vi "DJ Interface.vi"(10 "Owning VI":refnum<vi>, 11 "Shutdown Event":refnum<user-event>) -> ()   [LabVIEW 2018, in "User Interface.lvlib"]
doc: "Main control interface to Dataflow DJ. Also handles all keyboard shortcuts.\n\n<b>Execution System:</b> User Interface"
uses:
  User Interface.lvlib
  Custom Graphics/Slide.Vert.ctl
  Custom Graphics/LED.Red.16px.ctl
  Custom Graphics/Slide.Horiz.ctl
  Custom Graphics/Slide.PlaybackPosition.ctl
  Custom Graphics/WaveformGraph.WaveformDisplay.ctl
  Custom Graphics/Knob.276px_Hole.ctl
  Custom Graphics/Button.Large.ctl
  Custom Graphics/PictRing.DeckLabel.ctl
  Custom Graphics/Button.Small.ctl
  <vilib>/Utility/miscctls.llb/LVCursorListTypeDef.ctl
  Audio Processing/Value Properties.ctl
  Messaging/Message Cluster.ctl
  Controls/Keyboard Shortcut.ctl
  1bc07e46-b0f0-44a4-aabd-5c34d242854a.vi
  Messaging/Messaging.lvlib
  user32.dll
  Audio Processing/Audio Processing.lvlib
panel:
  in  "Mixer.Channel2.EQFilter":dbl(knob) scale=-1.025..1.025
  in  "Mixer.Channel1.EQFilter":dbl(knob) scale=-1.025..1.025
  in  "Deck2.DragDropPath":path
  in  "Deck1.DragDropPath":path
  in  "Deck1.Pitch":T1 scale=30.0..-30.0
  in  "Deck2.PitchBendUp":T2
  in  "Deck2.PitchBendDown":T2
  in  "Mixer.Channel2.HeadphoneOutput":T2
  in  "Mixer.Channel1.HeadphoneOutput":T2
  in  "Deck1.PitchBendUp":T2
  in  "Deck1.PitchBendDown":T2
  in  "Deck2.Reverse":T3
  in  "Deck2.Backspin":T3
  in  "Deck2.Brake":T3
  in  "Deck2.Cue3":T3
  in  "Deck2.Cue2":T3
  in  "Deck2.Cue1":T3
  in  "Deck2.Play":T3
  in  "Deck1.Cue3":T3
  in  "Deck1.Cue2":T3
  in  "Deck1.Reverse":T3
  in  "Deck1.Backspin":T3
  in  "Deck1.Cue1":T3
  out "Deck2.Time":string
  in  "Deck2.PlaybackPosition":T4 scale=0.0..7050240.0
  out "Deck2.Waveform":T5
  out "Deck2.BPM":string
  out "Deck1.BPM":string
  in  "Mixer.Headphones":dbl(knob)=1.0 scale=0.0..1.0
  in  "Deck1.Brake":T3
  in  "Mixer.Channel2.Effect3.Value2":dbl(knob) scale=0.0..1.0
  in  "Mixer.Channel2.Effect3.Enable":T6
  in  "Mixer.Channel2.Effect3.Value1":dbl(knob) scale=0.0..1.0
  in  "Mixer.Channel2.Effect2.Enable":T6
  in  "Mixer.Channel2.Effect2.Value1":dbl(knob)=1.0 step=1.0 scale=1.0..20.0
  in  "Mixer.Channel2.Effect2.Value2":dbl(knob)=16.0 step=1.0 scale=0.0..16.0
  in  "Mixer.Channel2.Effect1.Enable":T6
  in  "Mixer.Channel2.Effect1.Value1":dbl(knob) scale=0.0..1.0
  in  "Mixer.Channel2.Effect1.Value2":dbl(knob) scale=0.001..0.1
  in  "Mixer.Channel1.Effect3.Value2":dbl(knob) scale=0.0..1.0
  in  "Mixer.Channel1.Effect3.Enable":T6
  in  "Mixer.Channel1.Effect3.Value1":dbl(knob) scale=0.0..1.0
  out "Mixer.Channel2.LevelIndicator":u8(slide) scale=0.0..20.0
  out "Mixer.Channel1.LevelIndicator":u8(slide) scale=0.0..20.0
  in  "Mixer.Channel1.Effect2.Enable":T6
  in  "Mixer.Channel1.Effect2.Value1":dbl(knob)=1.0 step=1.0 scale=1.0..20.0
  in  "Mixer.Channel1.Effect2.Value2":dbl(knob)=16.0 step=1.0 scale=0.0..16.0
  in  "Mixer.Channel1.Effect1.Enable":T6
  in  "Deck1.Play":T3
  in  "Mixer.Master":dbl(knob)=1.0 scale=0.0..1.0
  in  "Deck1.Jogwheel":T7 scale=0.0..79380.0
  in  "Mixer.Channel1.Effect1.Value1":dbl(knob) scale=0.0..1.0
  in  "Mixer.Channel1.Effect1.Value2":dbl(knob) scale=0.001..0.1
  in  "Deck2.Pitch":T1 scale=30.0..-30.0
  out "Deck2.Title":string
  out "Deck1.Time":string
  out "Deck1.Title":string
  in  "Deck2.Jogwheel":T7 scale=0.0..79380.0
  in  "Mixer.Channel2.Level":T1=1.0 scale=0.0..1.0
  in  "Mixer.Channel2.EQHighKill":T6
  in  "Mixer.Channel2.EQMidKill":T6
  in  "Mixer.Channel2.EQLow":dbl(knob)=1.0 scale=0.0..2.0
  in  "Mixer.Channel2.EQMid":dbl(knob)=1.0 scale=0.0..2.0
  in  "Mixer.Channel2.EQHigh":dbl(knob)=1.0 scale=0.0..2.0
  in  "Mixer.Channel2.EQLowKill":T6
  in  "Mixer.Channel2.Gain":dbl(knob)=1.0 scale=0.0..2.0
  in  "Mixer.Crossfader":T8 scale=-1.0..1.0
  in  "Mixer.Channel1.Level":T1=1.0 scale=0.0..1.0
  in  "Mixer.Channel1.EQHighKill":T6
  in  "Mixer.Channel1.EQMidKill":T6
  in  "Mixer.Channel1.EQLow":dbl(knob)=1.0 scale=0.0..2.0
  in  "Mixer.Channel1.EQMid":dbl(knob)=1.0 scale=0.0..2.0
  in  "Mixer.Channel1.EQHigh":dbl(knob)=1.0 scale=0.0..2.0
  in  "Mixer.Channel1.EQLowKill":T6
  in  "Mixer.Channel1.Gain":dbl(knob)=1.0 scale=0.0..2.0
  in  "Deck1.PlaybackPosition":T4 scale=0.0..7050240.0
  out "Deck1.Waveform":T5
  out "Deck1.JogwheelLabel":T9
  out "Deck2.JogwheelLabel":T9
  # "GAIN"
  # "MASTER"
  # "PHONES"
  # "GAIN"
  # "FLANGER"
  # "FLANGER"
  # "AMOUNT"
  # "SPEED"
  # "AMOUNT"
  # "SPEED"
  # "CRUSHER"
  # "CRUSHER"
  # "DECIMATION"
  # "BIT DEPTH"
  # "DECIMATION"
  # "BIT DEPTH"
  # "ECHO"
  # "ECHO"
  # "AMOUNT"
  # "DELAY"
  # "AMOUNT"
  # "DELAY"
  # "DECK 1\nCUE"
  # "DECK 2\nCUE"
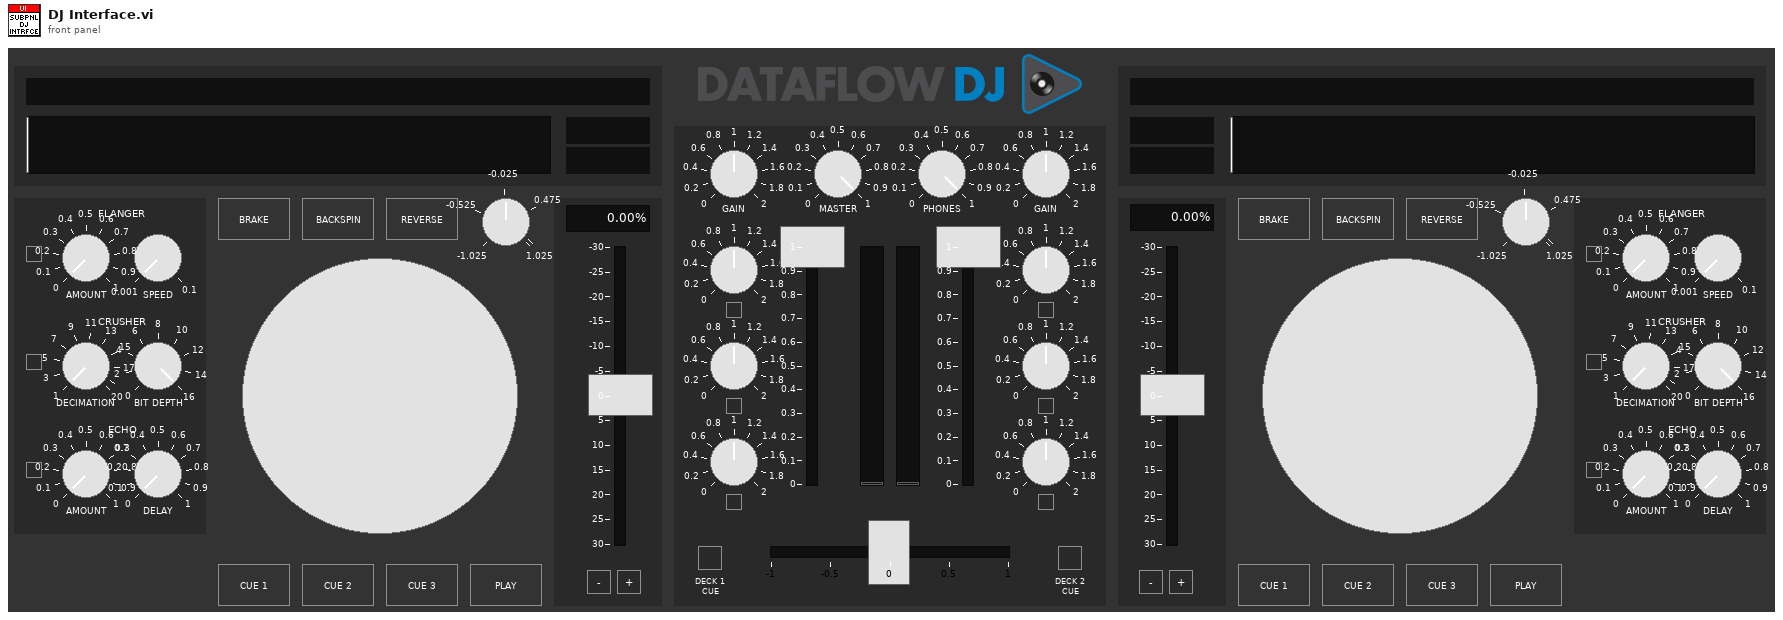
[diagram p1: front panel]
types:
  T1 = typedef "User Interface.lvlib/Slide.Vert.ctl" = dbl
  T2 = typedef "User Interface.lvlib/Button.Small.ctl" = bool
  T3 = typedef "User Interface.lvlib/Button.Large.ctl" = bool
  T4 = typedef "User Interface.lvlib/Slide.PlaybackPosition.ctl" = i32
  T5 = typedef "User Interface.lvlib/WaveformGraph.WaveformDisplay.ctl" = dbl[][]
  T6 = typedef "User Interface.lvlib/LED.Red.16px.ctl" = bool
  T7 = typedef "User Interface.lvlib/Knob.276px_Hole.ctl" = i32
  T8 = typedef "User Interface.lvlib/Slide.Horiz.ctl" = dbl
  T9 = typedef "User Interface.lvlib/PictRing.DeckLabel.ctl" = u16
  T10 = typedef "LVCursorListTypeDef.ctl" = cluster{"Name":string, "Color":u32, "Style":u8, "Point Style":u8, "Name Visible":bool, "Allow Drag":bool, "Cursor Mode":u32, "Plot":i32, "Index":i32, "Position":cluster{"X":dbl, "Y":dbl}, "X Scale":u32, "Y Scale":u32, "Watch Plots":i32[], "Watch All Plots":bool, "Plot Area":i32, "Label Offset":cluster{"X":dbl, "Y":dbl}}[]
  T11 = typedef "Keyboard Shortcut.ctl" = cluster{"Keystroke":string, "Message Queue":string, "Event":string, "Target":string, "Data":variant}
  T12 = typedef "Audio Processing.lvlib/Value Properties.ctl" = cluster{"Lower":dbl, "Upper":dbl}
  T13 = typedef "Messaging.lvlib/Message Cluster.ctl" = cluster{"Event":string, "Source":string, "Target":string, "Data":variant}
  T14 = cluster{"type":i32, "KEYBDINPUT":cluster{"dx":i32, "dy":i32, "mouseData":i32, "dwFlags":i32, "time":i32, "dwExtraInfo":u32}}
  T15 = typedef "eventvkey.ctl" = enum16{"ASCII", "Enter", "Return", "Shift", "Ctrl", "Alt", "Cmd", "Opt", "Caps", "NumLock", "Clear", "Break", "Up", "Down", "Left", "Right", "Insert", "Delete", "Home", "End", "PageUp", "PageDown", "Escape", "Help", "Pause", "ScrollLock", "F1", "F2", "F3", "F4", "F5", "F6", "F7", "F8", "F9", "F10", "F11", "F12", "F13", "F14", "F15", "F16", "F17", "F18", "F19", "F20", "F21", "F22", "F23", "F24", "Play", "VolumeUp", "VolumeDown", "Mute", "Two Byte Char"}
  T16 = cluster{"Shift":bool, "Ctrl":bool, "Alt":bool, "Cmd":bool, "Opt":bool}
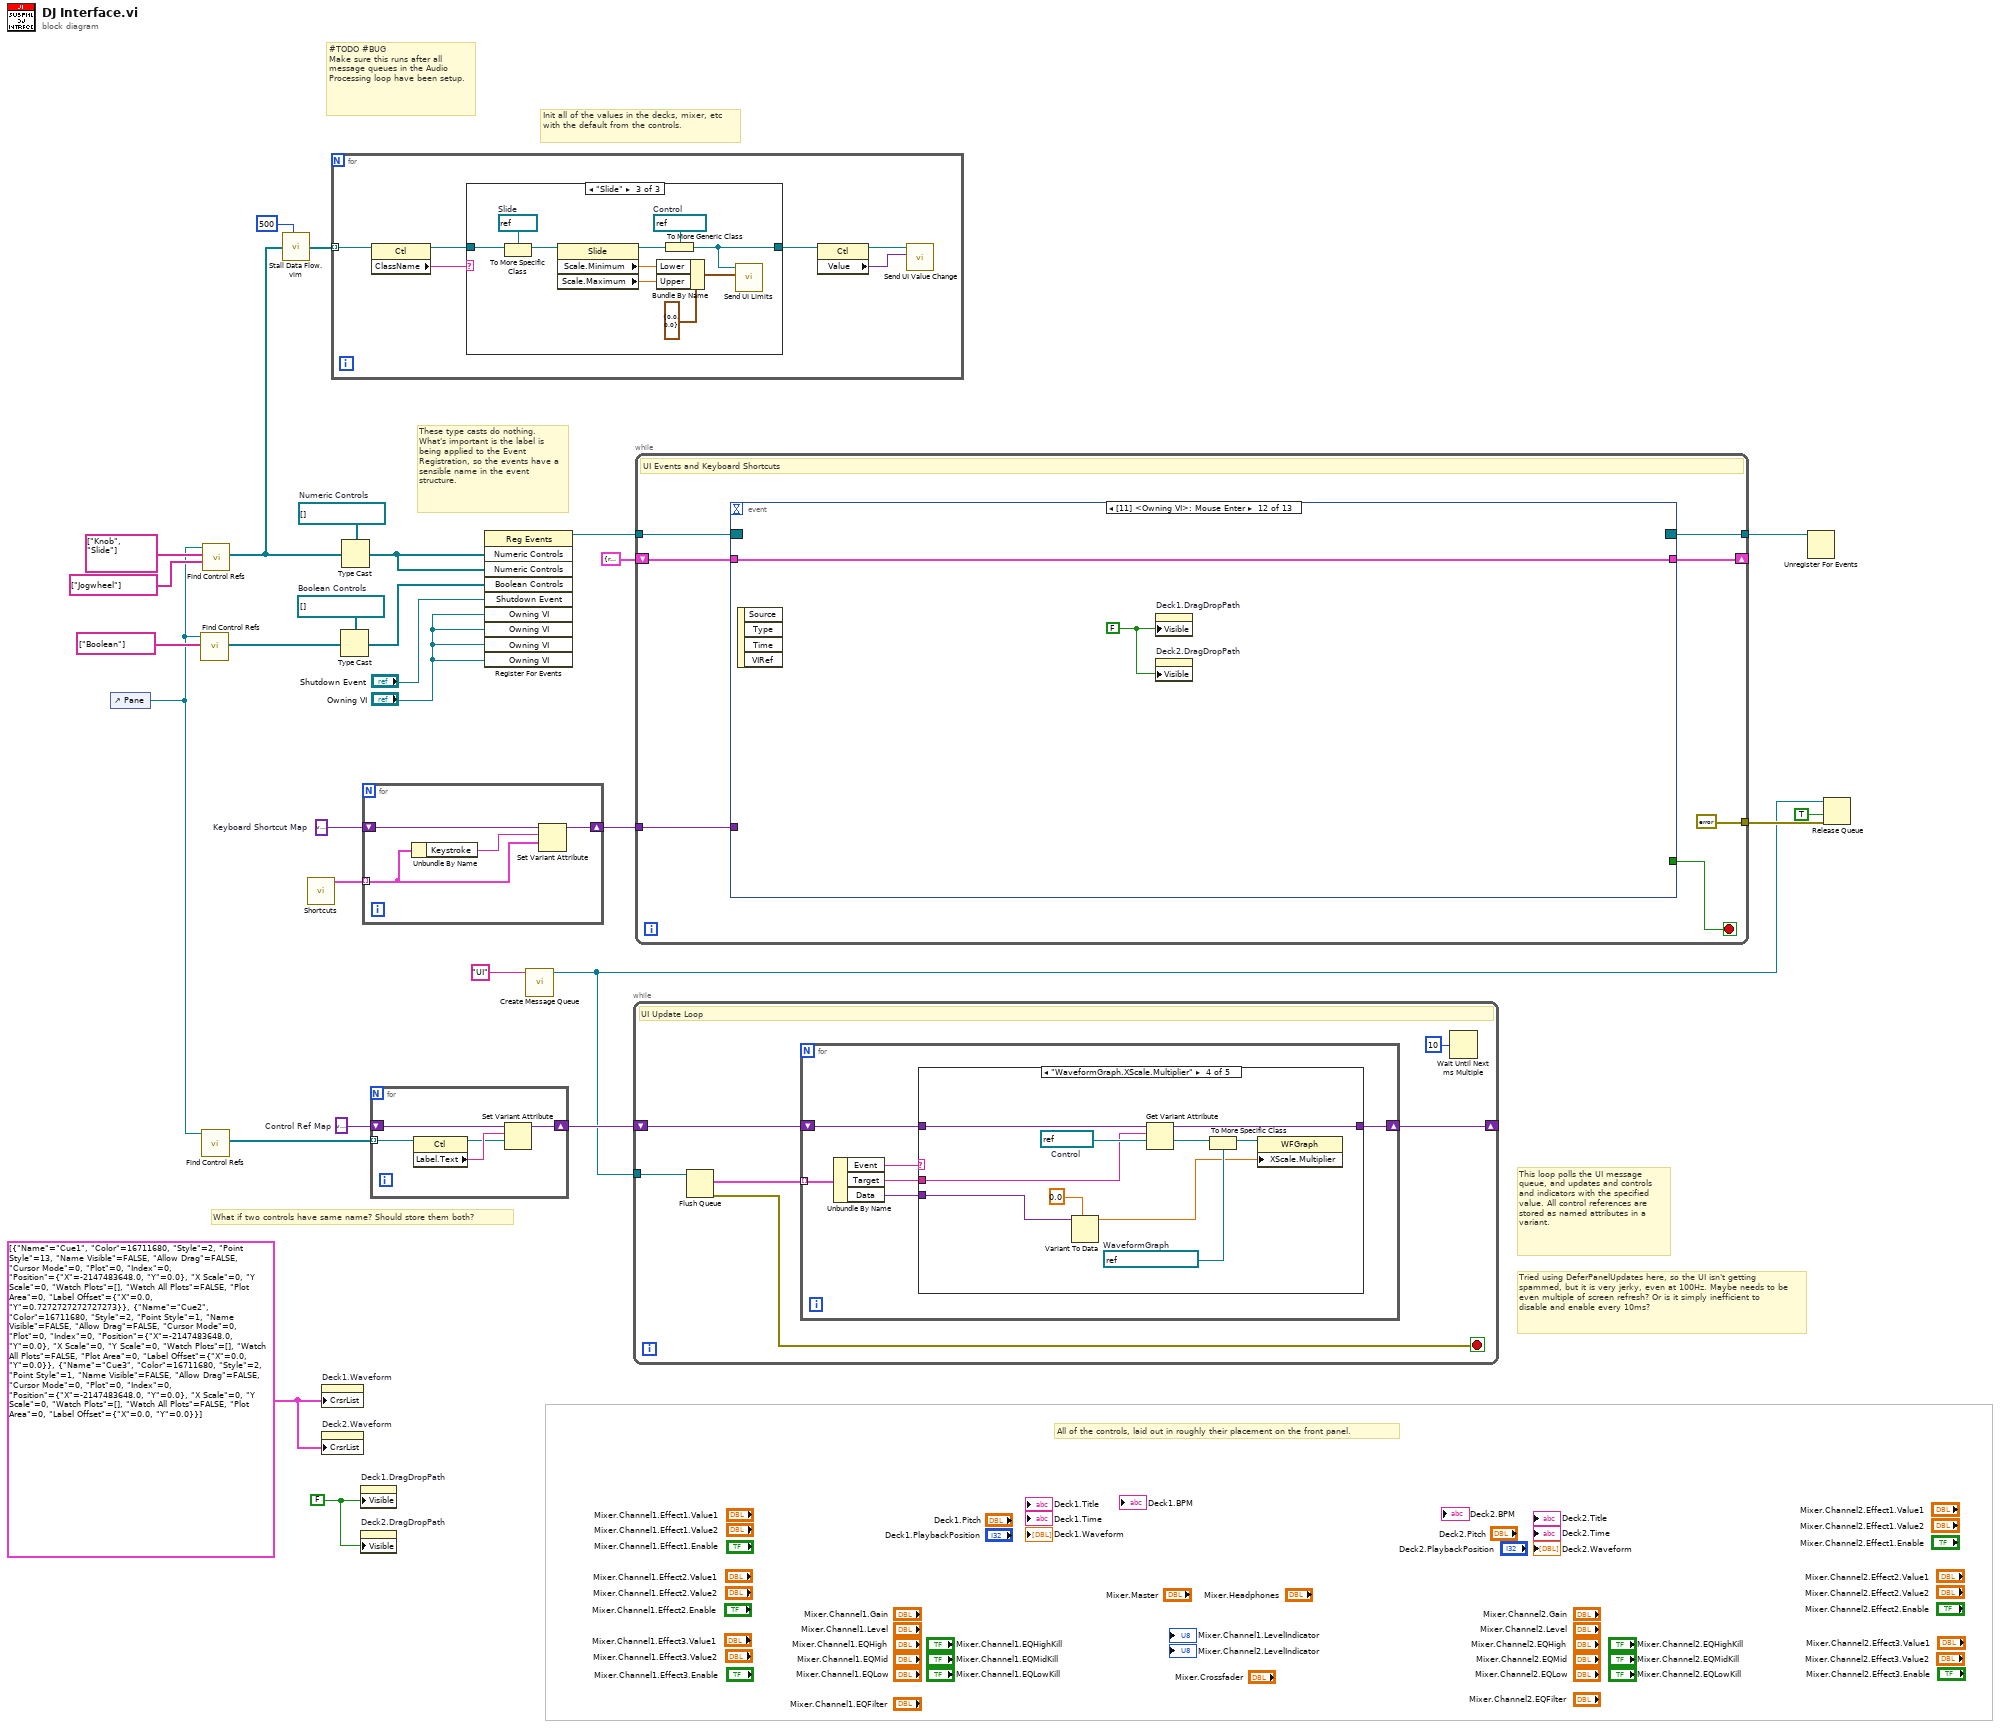
[diagram p0: block diagram]
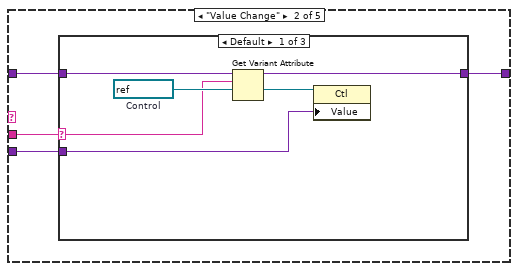
[diagram p3: hidden frame]
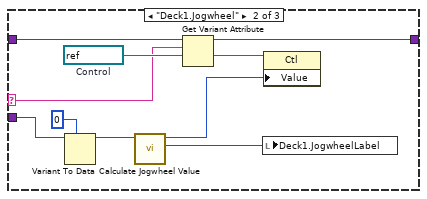
[diagram p4: hidden frame]
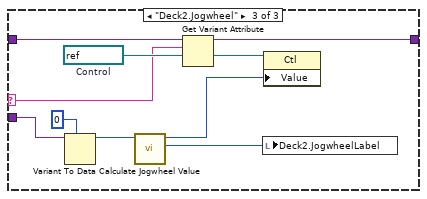
[diagram p5: hidden frame]
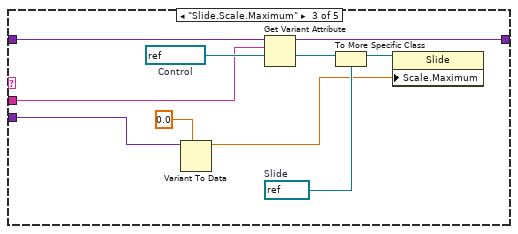
[diagram p6: hidden frame]
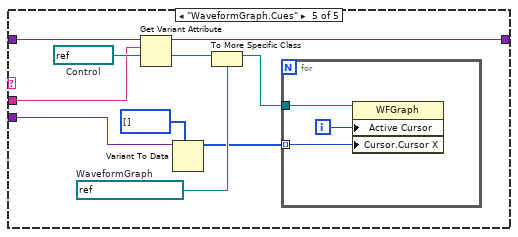
[diagram p7: hidden frame]
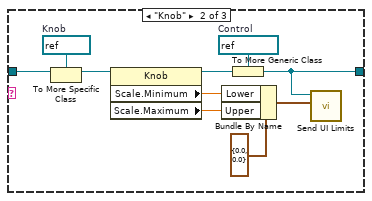
[diagram p9: hidden frame]
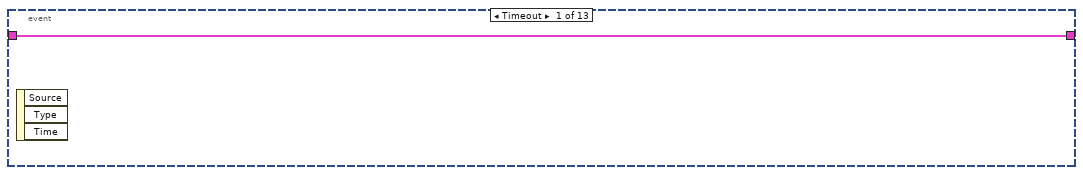
[diagram p10: hidden frame]
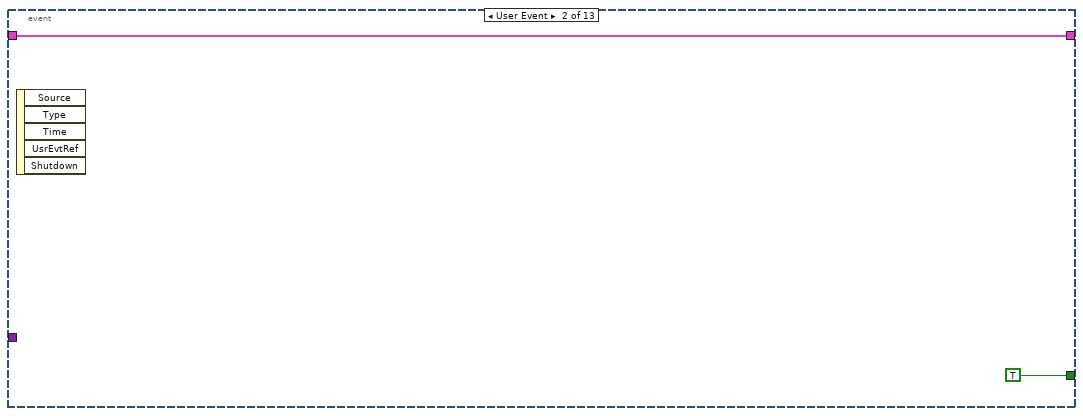
[diagram p11: hidden frame]
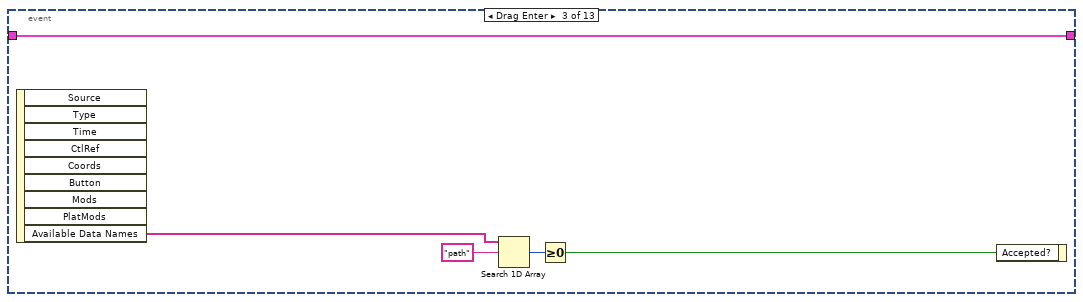
[diagram p12: hidden frame]
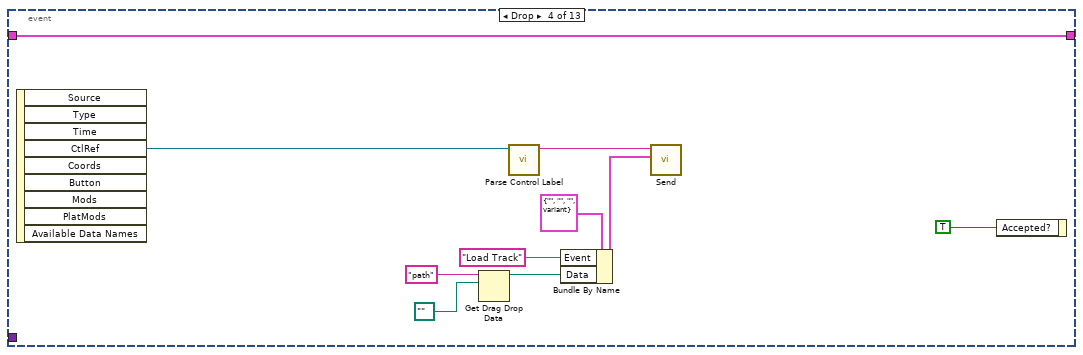
[diagram p13: hidden frame]
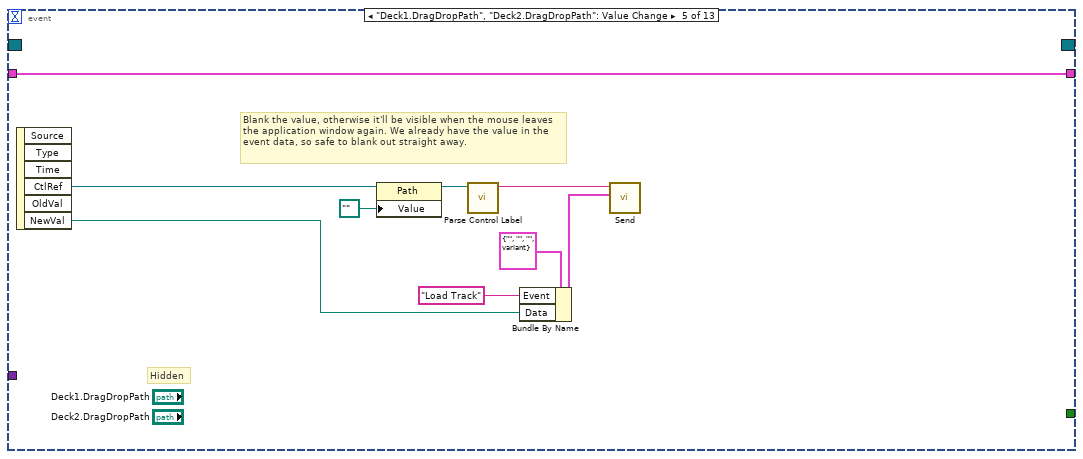
[diagram p14: hidden frame]
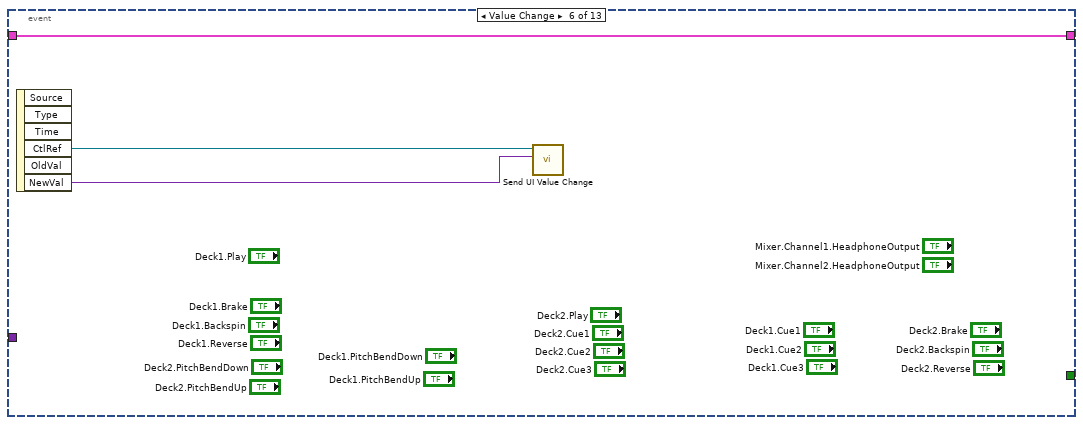
[diagram p15: hidden frame]
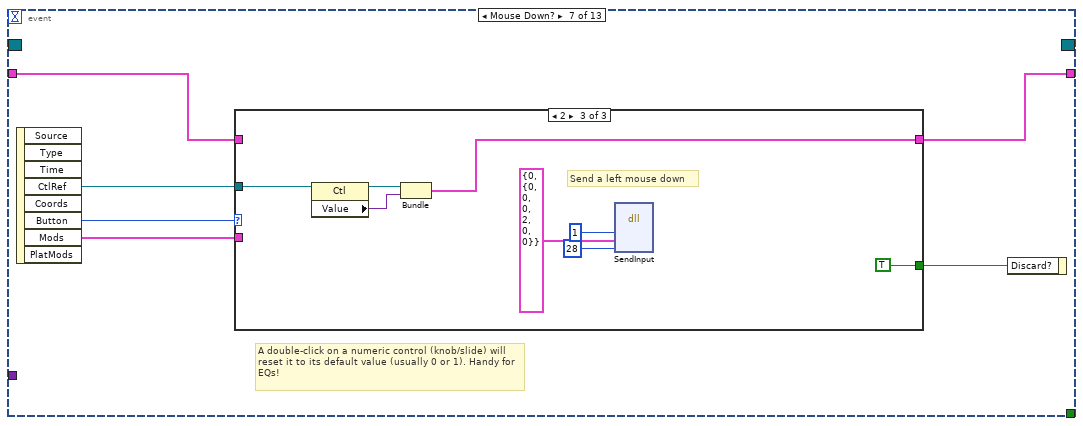
[diagram p16: hidden frame]
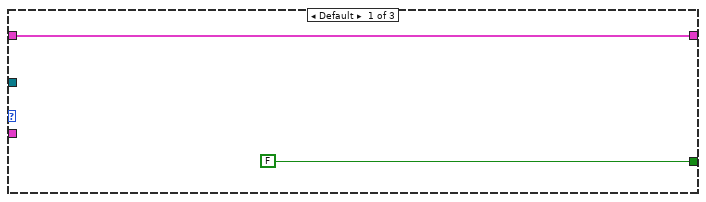
[diagram p17: hidden frame]
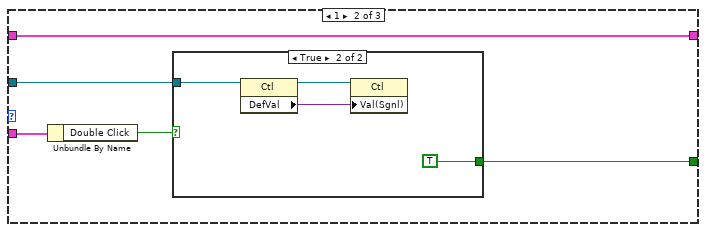
[diagram p18: hidden frame]
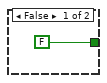
[diagram p19: hidden frame]
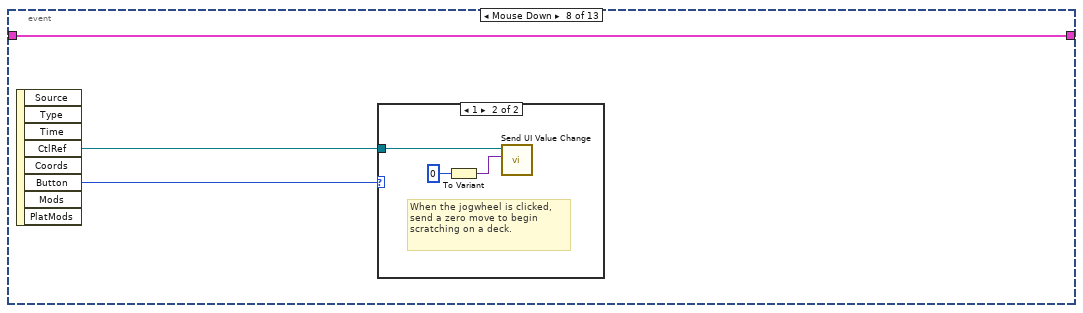
[diagram p20: hidden frame]
diagram:
  w4 = FALSE ("Visible")
  w6 = T10 [{"Name"="Cue1", "Color"=16711680, "Style"=2, "Point Style"=13, "Name Visible"=FALSE, "Allow Drag"=FALSE, "Cursor Mode"=0, "Plot"=0, "Index"=0, "Position"={"X"=-2147483648.0, "Y"=0.0}, "X Scale"=0, "Y Scale"=0, "Watch Plots"=[], "Watch All Plots"=FALSE, "Plot Area"=0, "Label Offset"={"X"=0.0, "Y"=0.7272727272727273}}, {"Name"="Cue2", "Color"=16711680, "Style"=2, "Point Style"=1, "Name Visible"=FALSE, "Allow Drag"=FALSE, "Cursor Mode"=0, "Plot"=0, "Index"=0, "Position"={"X"=-2147483648.0, "Y"=0.0}, "X Scale"=0, "Y Scale"=0, "Watch Plots"=[], "Watch All Plots"=FALSE, "Plot Area"=0, "Label Offset"={"X"=0.0, "Y"=0.0}}, {"Name"="Cue3", "Color"=16711680, "Style"=2, "Point Style"=1, "Name Visible"=FALSE, "Allow Drag"=FALSE, "Cursor Mode"=0, "Plot"=0, "Index"=0, "Position"={"X"=-2147483648.0, "Y"=0.0}, "X Scale"=0, "Y Scale"=0, "Watch Plots"=[], "Watch All Plots"=FALSE, "Plot Area"=0, "Label Offset"={"X"=0.0, "Y"=0.0}}] ("Cursor List")
  w21 = variant  # Keyboard Shortcut Map
  w24 = variant  # Control Ref Map
  w28 = refnum<vi>[] []  # Boolean Controls
  w27 = refnum<vi>[] []  # Numeric Controls
  # "Init all of the values in the decks, mixer, etc with the default from the controls."
  # "#TODO #BUG\nMake sure this runs after all message queues in the Audio Processing loop have been setup."
  # "What if two controls have same name? Should store them both?"
  # "All of the controls, laid out in roughly their placement on the front panel."
  # "This loop polls the UI message queue, and updates and controls and indicators with the specified value. All control references are stored as named attributes in a variant."
  # "Tried using DeferPanelUpdates here, so the UI isn't getting spammed, but it is very jerky, even at 100Hz. Maybe needs to be even multiple of screen refresh? Or is it simply inefficient to disable and enable every 10ms?"
  # "These type casts do nothing. What's important is the label is being applied to the Event Registration, so the events have a sensible name in the event structure."
  n1 = control-ref of="Pane"() -> (w10:refnum<vi>)
  n2 = call "Find Control Refs.vi"("Control Types"=string[] ["Boolean"], "Pane Reference In"=w10) -> ("Control Refs"=w11:refnum<vi>[])  [unwired: 8 in, 1 out]
  n3 = call "Find Control Refs.vi"("Pane Reference In"=w10) -> ("Control Refs"=w9:refnum<vi>[])  [unwired: 9 in, 1 out]
  n4 = call "Find Control Refs.vi"("Label.Text Filter"=string[] ["Jogwheel"], "Control Types"=string[] ["Knob", "Slide"], "Pane Reference In"=w10) -> ("Control Refs"=w3:refnum<vi>[])  [unwired: 7 in, 1 out]
  n5 = call "Stall Data Flow.vim"("value in"=w3, "milliseconds to wait"=u32 500) -> ("value out"=w2:refnum<vi>[])  [unwired: 1 out]
  n6 = call "Shortcuts.vi"() -> ("Keyboard Shortcuts"=w19:T11[])  [unwired: 11 in]
  n7 = property on="Deck1.Waveform" class="WFGraph (strict)"("CrsrList"=w6) -> ()  [unwired: 2 in, 2 out]
  n8 = property on="Deck2.Waveform" class="WFGraph (strict)"("CrsrList"=w6) -> ()  [unwired: 2 in, 2 out]
  n9 = for {
    tunnel: w2 -> [w31] mode=indexing
    n10 = property class="Ctl"(reference=w31) -> (reference out=w32:refnum<vi>, "ClassName"=w30:string)  [unwired: 1 in, 1 out]
    n11 = case shown="\"Slide\"" w30 {
      tunnel: [w36 w41 w48] -> w33
      tunnel: w32 -> [w36 w46 w56]
      frame Default {
      }
      frame "Knob" {
        w42 = refnum<vi> refnum  # Control
        w45 = refnum<vi> refnum  # Knob
        n12 = To More Specific Class(target class=w45, reference=w46) -> (specific class reference=w44:refnum<vi>)  [unwired: 1 in, 1 out]
        n13 = property class="Knob"(reference=w44) -> (reference out=w43:refnum<vi>, "Scale.Minimum"=w39:dbl, "Scale.Maximum"=w38:dbl)  [unwired: 1 in, 1 out]
        n14 = Bundle By Name(cluster=T12 {"Lower"=0.0, "Upper"=0.0} ("Value Properties"), "Lower"=w39, "Upper"=w38) -> (w37:T12)
        n15 = To More Generic Class(target class=w42, reference=w43) -> (generic class reference=w41:refnum<vi>)
        n16 = call "Send UI Limits.vi"("Data"=w37, "CtlRef"=w41) -> ()  [unwired: 10 in]
      }
      frame "Slide" {
        w49 = refnum<vi> refnum  # Control
        w55 = refnum<vi> refnum  # Slide
        n17 = To More Specific Class(target class=w55, reference=w56) -> (specific class reference=w54:refnum<vi>)  [unwired: 1 in, 1 out]
        n18 = property class="Slide"(reference=w54) -> (reference out=w50:refnum<vi>, "Scale.Minimum"=w53:dbl, "Scale.Maximum"=w52:dbl)  [unwired: 1 in, 1 out]
        n19 = Bundle By Name(cluster=T12 {"Lower"=0.0, "Upper"=0.0} ("Value Properties"), "Lower"=w53, "Upper"=w52) -> (w51:T12)
        n20 = To More Generic Class(target class=w49, reference=w50) -> (generic class reference=w48:refnum<vi>)
        n21 = call "Send UI Limits.vi"("Data"=w51, "CtlRef"=w48) -> ()  [unwired: 10 in]
      }
    }
    n22 = property class="Ctl"(reference=w33) -> (reference out=w34:refnum<vi>, "Value"=w35:variant)  [unwired: 1 in, 1 out]
    n23 = call "Send UI Value Change.vi"("Data"=w35, "CtlRef"=w34) -> ()  [unwired: 10 in]
  }
  n24 = Type Cast(type=w28, x=w11) -> (*(type *) &x=w25:refnum<vi>[])
  n25 = Type Cast(type=w27, x=w3) -> (*(type *) &x=w8:refnum<vi>[])
  n26 = property on="Deck1.DragDropPath" class="Path"("Visible"=w4) -> ()  [unwired: 2 in, 2 out]
  n27 = property on="Deck2.DragDropPath" class="Path"("Visible"=w4) -> ()  [unwired: 2 in, 2 out]
  n28 = for {
    shift-right: [w59] -> w20
    shift-left: w21 -> [w60]
    tunnel: w19 -> [w57] mode=indexing
    n29 = Unbundle By Name(w57) -> ("Keystroke"=w58:string)
    n30 = Set Variant Attribute(Variant=w60, name=w58, value=w57) -> (Variant out=w59:variant)  [unwired: 1 in, 2 out]
  }
  n31 = for {
    shift-right: [w64] -> w23
    shift-left: w24 -> [w65]
    tunnel: w9 -> [w63] mode=indexing
    n32 = property class="Ctl"(reference=w63) -> (reference out=w61:refnum<vi>, "Label.Text"=w62:string)  [unwired: 1 in, 1 out]
    n33 = Set Variant Attribute(Variant=w65, name=w62, value=w61) -> (Variant out=w64:variant)  [unwired: 1 in, 2 out]
  }
  n34 = register-events(w8, w8, w25, "Shutdown Event", "Owning VI", "Owning VI", "Owning VI", "Owning VI") -> (reference out=w29:refnum<event-registration>)  [unwired: 2 in, 1 out]
  n35 = call "Create Message Queue.vi"("Queue Name"="UI") -> ("queue out"=w15:refnum<queue>)  [unwired: 9 in, 1 out]
  n36 = while {
    tunnel: w15 -> [w69]
    shift-right: [w70] -> _
    shift-left: w23 -> [w71]
    stop <- w67 stop-if-true
    # "UI Update Loop"
    n37 = Flush Queue(queue=w69) -> (remaining elements=w66:T13[], error out=w67:errorcluster)  [unwired: 1 in, 1 out]
    n38 = for {
      shift-right: [w76] -> w70
      shift-left: w71 -> [w77]
      tunnel: w66 -> [w72] mode=indexing
      n39 = Unbundle By Name(w72) -> ("Event"=w75:string, "Target"=w73:string, "Data"=w74:variant)
      n40 = case shown="\"WaveformGraph.XScale.Multiplier\"" w75 {
        tunnel: w77 -> [w78 w82 w118 w128 w138]
        tunnel: w73 -> [_ w79 w115 w125 w135]
        tunnel: [w78 w81 w116 w126 w136] -> w76
        tunnel: w74 -> [_ w80 w110 w120 w130]
        frame Default {
        }
        frame "Value Change" {
          n41 = case shown="Default" w79 {
            selector: w79 -> [w83 w94 w104]
            tunnel: w82 -> [w88 w98 w108]
            tunnel: [w85 w95 w105] -> w81
            tunnel: w80 -> [w84 w93 w103]
            frame Default {
              w87 = refnum<vi> refnum  # Control
              n42 = Get Variant Attribute(Variant=w88, name=w83, default value (empty Variant)=w87) -> (duplicate Variant=w85:variant, value=w86:refnum<vi>)  [unwired: 1 in, 2 out]
              n43 = property class="Ctl"(reference=w86, "Value"=w84) -> ()  [unwired: 1 in, 2 out]
            }
            frame "Deck1.Jogwheel" {
              w97 = refnum<vi> refnum  # Control
              n44 = Variant To Data(type=0 ("y"), Variant=w93) -> (data=w91:i32)  [unwired: 1 in, 1 out]
              n45 = call "Calculate Jogwheel Value.vi"("Playback Position"=w91) -> ("Jogwheel Label Image"=w89:i32, "Jogwheel Position"=w90:i32)  [unwired: 9 in]
              n46 = Get Variant Attribute(Variant=w98, name=w94, default value (empty Variant)=w97) -> (duplicate Variant=w95:variant, value=w96:refnum<vi>)  [unwired: 1 in, 2 out]
              n47 = local write "Deck1.JogwheelLabel"(w89) -> ()
              n48 = property class="Ctl"(reference=w96, "Value"=w90) -> ()  [unwired: 1 in, 2 out]
            }
            frame "Deck2.Jogwheel" {
              w107 = refnum<vi> refnum  # Control
              n49 = Variant To Data(type=0 ("y"), Variant=w103) -> (data=w101:i32)  [unwired: 1 in, 1 out]
              n50 = call "Calculate Jogwheel Value.vi"("Playback Position"=w101) -> ("Jogwheel Label Image"=w99:i32, "Jogwheel Position"=w100:i32)  [unwired: 9 in]
              n51 = Get Variant Attribute(Variant=w108, name=w104, default value (empty Variant)=w107) -> (duplicate Variant=w105:variant, value=w106:refnum<vi>)  [unwired: 1 in, 2 out]
              n52 = local write "Deck2.JogwheelLabel"(w99) -> ()
              n53 = property class="Ctl"(reference=w106, "Value"=w100) -> ()  [unwired: 1 in, 2 out]
            }
          }
        }
        frame "Slide.Scale.Maximum" {
          w114 = refnum<vi> refnum  # Slide
          w117 = refnum<vi> refnum  # Control
          n54 = Variant To Data(type=0.0, Variant=w110) -> (data=w111:dbl)  [unwired: 1 in, 1 out]
          n55 = Get Variant Attribute(Variant=w118, name=w115, default value (empty Variant)=w117) -> (duplicate Variant=w116:variant, value=w113:refnum<vi>)  [unwired: 1 in, 2 out]
          n56 = To More Specific Class(target class=w114, reference=w113) -> (specific class reference=w112:refnum<vi>)  [unwired: 1 in, 1 out]
          n57 = property class="Slide"(reference=w112, "Scale.Maximum"=w111) -> ()  [unwired: 1 in, 2 out]
        }
        frame "WaveformGraph.XScale.Multiplier" {
          w124 = refnum<vi> refnum  # WaveformGraph
          w127 = refnum<vi> refnum  # Control
          n58 = Variant To Data(type=0.0, Variant=w120) -> (data=w121:dbl)  [unwired: 1 in, 1 out]
          n59 = Get Variant Attribute(Variant=w128, name=w125, default value (empty Variant)=w127) -> (duplicate Variant=w126:variant, value=w123:refnum<vi>)  [unwired: 1 in, 2 out]
          n60 = To More Specific Class(target class=w124, reference=w123) -> (specific class reference=w122:refnum<vi>)  [unwired: 1 in, 1 out]
          n61 = property class="WFGraph"(reference=w122, "XScale.Multiplier"=w121) -> ()  [unwired: 1 in, 2 out]
        }
        frame "WaveformGraph.Cues" {
          w134 = refnum<vi> refnum  # WaveformGraph
          w137 = refnum<vi> refnum  # Control
          n62 = Get Variant Attribute(Variant=w138, name=w135, default value (empty Variant)=w137) -> (duplicate Variant=w136:variant, value=w133:refnum<vi>)  [unwired: 1 in, 2 out]
          n63 = Variant To Data(type=i32[] [], Variant=w130) -> (data=w131:i32[])  [unwired: 1 in, 1 out]
          n64 = To More Specific Class(target class=w134, reference=w133) -> (specific class reference=w132:refnum<vi>)  [unwired: 1 in, 1 out]
          n65 = for {
            tunnel: w132 -> [w141]
            tunnel: w131 -> [w140] mode=indexing
            i -> [w139]
            n66 = property class="WFGraph"(reference=w141, "Active Cursor"=w139, "Cursor.Cursor X"=w140) -> ()  [unwired: 1 in, 2 out]
          }
        }
      }
    }
    n67 = Wait Until Next ms Multiple(millisecond multiple=u32 10) -> ()  [unwired: 1 out]
  }
  n68 = while {
    tunnel: [errorcluster {"status"=FALSE, "code"=0, "source"=""} ("error in (no error)")] -> w22
    tunnel: w29 -> [w147]
    tunnel: [w146] -> w26
    tunnel: w20 -> [w145]
    shift-right: [w143] -> _
    shift-left: cluster{"CtlRef":refnum<vi>, "Value":variant} {"CtlRef"=refnum, "Value"=variant} -> [w142]
    stop <- w144 stop-if-true
    # "UI Events and Keyboard Shortcuts"
    n69 = event shown="[11] <Owning VI>: Mouse Enter" {
      selector: w147 -> [_ _ _ _ _ _ _ _ _ _ _ _ _]
      dyn-events: [_ _ _ _ _ _ _ _ _ _ _ _ _] -> w146
      timeout: _ -> [_ _ _ _ _ _ _ _ _ _ _ _ _]
      tunnel: w145 -> [_ _ _ _ _ _ _ _ _ w227 _ _ _]
      tunnel: [_ TRUE _ _ _ _ _ _ _ _ _ _ _] -> w144
      tunnel: [w149 w150 w152 w157 w175 w176 w180 w205 w211 w221 w240 w261 w263] -> w143
      tunnel: w142 -> [w149 w150 w152 w157 w175 w176 w179 w205 w211 w221 w241 w261 w263]
      event Timeout {
        n70 = event-data() -> ()  [unwired: 1 in, 3 out]
      }
      event User Event {
        n71 = event-data() -> ()  [unwired: 1 in, 5 out]
      }
      event Drag Enter {
        n72 = event-data() -> ("Available Data Names"=w154:string[])  [unwired: 1 in, 8 out]
        n73 = Search 1D Array(1D array=w154, element="path") -> (index of element=w155:i32)  [unwired: 1 in]
        n74 = Greater Or Equal To 0?(x=w155) -> (x >= 0?=w153:bool)
        n75 = event-data("Accepted?"=w153) -> ()  [unwired: 1 in, 1 out]
      }
      event Drop {
        n76 = event-data() -> ("CtlRef"=w160:refnum<vi>)  [unwired: 1 in, 8 out]
        n77 = Get Drag Drop Data(8:path "", 9:"path" ("data name")) -> (3:w158:path)  [unwired: 1 in, 1 out]
        n78 = call "Parse Control Label.vi"("CtlRef"=w160) -> ("Queue Name"=w159:string)  [unwired: 9 in, 1 out]
        n79 = Bundle By Name(cluster=T13 {"Event"="", "Source"="", "Target"="", "Data"=variant} ("Message"), "Event"="Load Track" ("Type"), "Data"=w158) -> (w162:T13)
        n80 = call "Send.vi"("Message"=w162, "Queue Name"=w159) -> ()  [unwired: 9 in, 1 out]
        n81 = event-data("Accepted?"=TRUE) -> ()  [unwired: 1 in, 1 out]
      }
      event "Deck1.DragDropPath", "Deck2.DragDropPath": Value Change {
        # "Hidden"
        # "Blank the value, otherwise it'll be visible when the mouse leaves the application window again. We already have the value in the event data, so safe to blank out straight away."
        n82 = event-data() -> ("CtlRef"=w169:refnum<vi>, "NewVal"=w170:path)  [unwired: 1 in, 4 out]
        n83 = property class="Path"(reference=w169, "Value"=path "") -> (reference out=w167:refnum<vi>)  [unwired: 1 in, 1 out]
        n84 = call "Parse Control Label.vi"("CtlRef"=w167) -> ("Queue Name"=w174:string)  [unwired: 9 in, 1 out]
        n85 = Bundle By Name(cluster=T13 {"Event"="", "Source"="", "Target"="", "Data"=variant} ("Message"), "Event"="Load Track" ("Type"), "Data"=w170) -> (w172:T13)
        n86 = call "Send.vi"("Message"=w172, "Queue Name"=w174) -> ()  [unwired: 9 in, 1 out]
      }
      event Value Change {
        n87 = event-data() -> ("CtlRef"=w178:refnum<vi>, "NewVal"=w177:variant)  [unwired: 1 in, 4 out]
        n88 = call "Send UI Value Change.vi"("Data"=w177, "CtlRef"=w178) -> ()  [unwired: 10 in]
      }
      event Mouse Down? {
        # "A double-click on a numeric control (knob/slide) will reset it to its default value (usually 0 or 1). Handy for EQs!"
        n89 = event-data() -> ("CtlRef"=w182:refnum<vi>, "Button"=w184:u16, "Mods"=w183:cluster{"Double Click":bool, "Menu Key":bool})  [unwired: 1 in, 5 out]
        n90 = case shown="2" w184 {
          tunnel: w183 -> [_ w191 _]
          tunnel: w182 -> [_ w190 w200]
          tunnel: [FALSE ("Discard?") w188 TRUE ("Discard?")] -> w181
          tunnel: [w185 w187 w197] -> w180
          tunnel: w179 -> [w185 w187 _]
          frame Default {
          }
          frame 1 {
            n91 = Unbundle By Name(w191) -> ("Double Click"=w189:bool)
            n92 = case shown="True" w189 {
              tunnel: w190 -> [_ w195]
              tunnel: [FALSE ("Discard?") TRUE ("Discard?")] -> w188
              frame False {
              }
              frame True {
                n93 = property class="Ctl"(reference=w195) -> (reference out=w196:refnum<vi>, "DefVal"=w194:variant)  [unwired: 1 in, 1 out]
                n94 = property class="Ctl"(reference=w196, "Val(Sgnl)"=w194) -> ()  [unwired: 1 in, 2 out]
              }
            }
          }
          frame 2 {
            # "Send a left mouse down"
            n95 = property class="Ctl"(reference=w200) -> (reference out=w199:refnum<vi>, "Value"=w198:variant)  [unwired: 1 in, 1 out]
            n96 = Bundle("CtlRef"=w199, "Value"=w198) -> (w197:cluster{"CtlRef":refnum<vi>, "Value":variant})  [unwired: 1 in]
            n97 = dll-call lib="user32.dll" fn="SendInput"("nInputs"=u32 1, "pInputs"=T14 {"type"=0, "KEYBDINPUT"={"dx"=0, "dy"=0, "mouseData"=0, "dwFlags"=2, "time"=0, "dwExtraInfo"=0}} ("input"), "cbSize"=u32 28) -> ()  [unwired: 7 in, 2 out]
          }
        }
        n98 = event-data("Discard?"=w181) -> ()  [unwired: 1 in, 1 out]
      }
      event Mouse Down {
        n99 = event-data() -> ("CtlRef"=w207:refnum<vi>, "Button"=w206:u16)  [unwired: 1 in, 6 out]
        n100 = case shown="1" w206 {
          tunnel: w207 -> [_ w210]
          frame Default {
          }
          frame 1 {
            # "When the jogwheel is clicked, send a zero move to begin scratching on a deck."
            n101 = To Variant(anything=0) -> (Variant=w208:variant)
            n102 = call "Send UI Value Change.vi"("Data"=w208, "CtlRef"=w210) -> ()  [unwired: 10 in]
          }
        }
      }
      event Value Change {
        n103 = event-data() -> ("CtlRef"=w213:refnum<vi>, "OldVal"=w217:T7, "NewVal"=w216:T7)  [unwired: 1 in, 3 out]
        n104 = call "Calculate Jogwheel Value.vi"("Playback Position"=w216) -> ("Jogwheel Label Image"=w218:i32)  [unwired: 9 in, 1 out]
        n105 = call "Calculate Jogwheel Delta.vi"("New Value"=w216, "Old Value"=w217) -> ("Delta Value"=w215:i32)  [unwired: 9 in]
        n106 = To Variant(anything=w215) -> (Variant=w214:variant)
        n107 = call "Send UI Value Change.vi"("Data"=w214, "CtlRef"=w213) -> ()  [unwired: 10 in]
        n108 = call "Parse Control Label.vi"("CtlRef"=w213) -> ("Queue Name"=w212:string)  [unwired: 9 in, 1 out]
        n109 = case shown="\"Deck2\"" w212 {
          tunnel: w218 -> [_ w219 w220]
          frame Default {
          }
          frame "Deck1" {
            "Deck1.JogwheelLabel" <- w219
          }
          frame "Deck2" {
            "Deck2.JogwheelLabel" <- w220
          }
        }
      }
      event Key Down?; event type 5.0.x8000000b; event type 1.0.x8000000b {
        # "Register Key Down events on both THIS VI (running in a sub panel), and the owning VI. Why both? Why not just the owning VI?\n\nUsing just the Key Down event from the owning VI works, EXCEPT for when the mouse is being held down at the same time. LabVIEW seems to redirect all input focus to the sub panel VI (this VI) while the mouse button is being held. As such the owning VI can no longer generate Key Down events."
        # "#BUG\nWhile holding the mouse button down on a control (moving a slider for example), F10 will not register as a key press. All other function keys seem to work.\n\nWTF.\n\nHelp mentions F3 being an issue, but that's always worked. F1 will trigger the LabVIEW help if the key press isn't discarded."
        # "#TODO\nIf file browser controls are in focus, don't execute shortcuts? Or at least allow certain key presses (arrow keys, pgup, pgdwn, home, end, etc)"
        # "Always discard the key press, and don't pass them on to controls or LabVIEW itself."
        # "Keyboard shortcuts can be setup directly on a control, but LabVIEW only supports function keys and other non-ASCII inputs. In this case we want any key to be a possible shortcut, so all key presses are captured here."
        n110 = event-data() -> ("VKey"=w223:T15, "ScanCode"=w224:i16, "Mods"=w225:cluster{"Num Pad":bool, "Menu Key":bool}, "PlatMods"=w226:T16)  [unwired: 1 in, 6 out]
        n111 = call "Parse Key Press.vi"("PlatMods"=w226, "Mods"=w225, "ScanCode"=w224, "VKey"=w223) -> ("Key Pressed"=w228:string)  [unwired: 7 in]
        n112 = Get Variant Attribute(Variant=w227, name=w228, default value (empty Variant)=T11 {"Keystroke"="", "Message Queue"="", "Event"="", "Target"="", "Data"=variant(bool FALSE)}) -> (found=w230:bool, value=w229:T11)  [unwired: 1 in, 2 out]
        n113 = case shown="True" w230 {
          tunnel: w229 -> [_ w239]
          frame False {
          }
          frame True {
            n114 = Unbundle By Name(w239) -> ("Message Queue"=w238:string, "Event"=w235:string, "Target"=w234:string, "Data"=w232:variant)
            n115 = Bundle By Name(cluster=T13 {"Event"="", "Source"="", "Target"="", "Data"=variant} ("Message"), "Event"=w235, "Target"=w234, "Data"=w232, "Source"="Shortcut") -> (w236:T13)
            n116 = call "Send.vi"("Message"=w236, "Queue Name"=w238) -> ()  [unwired: 9 in, 1 out]
          }
        }
        n117 = event-data("Discard?"=TRUE) -> ()  [unwired: 1 in, 1 out]
      }
      event Mouse Up {
        # "#NOTE\nAny changes here should be duplicated in the Mouse Up (Outside Pane) user event."
        # "Possible #BUG ?\nIf a left-mouse down is being simulated (via a right-click on a numeric), and then the right-mouse is released, a left-mouse up is simulated. LabVIEW then receives that left-mouse up and processes the command here.\n\nCould have a flag to indicate the left mouse up was simulated and ignore it?"
        n118 = event-data() -> ("Button"=w242:u16)  [unwired: 1 in, 7 out]
        n119 = case shown="1" w242 {
          tunnel: w241 -> [w243 w249 w253]
          tunnel: [w243 w249 cluster{"CtlRef":refnum<vi>, "Value":variant} {"CtlRef"=refnum, "Value"=variant}] -> w240
          frame Default {
          }
          frame 1 {
            # "#TODO\nPoll mouse buttons using Input Device Control for mouse up instead?"
            # "The Mouse Up event is sent to each deck to cancel a scratch.\n\nNote that the Mouse Up is for the entire pane (not just a jogwheel) as the mouse will more than likely NOT be over the jogwheel. This doesn't help the case where the mouse is released outside the window entirely."
            n120 = Bundle By Name(cluster=T13 {"Event"="", "Source"="", "Target"="", "Data"=variant} ("Message"), "Event"="Mouse Up" ("Type")) -> (w244:T13)
            n121 = call "Send.vi"("Message"=w244, "Queue Name"="Deck1") -> ()  [unwired: 9 in, 1 out]
            n122 = call "Send.vi"("Message"=w244, "Queue Name"="Deck2") -> ()  [unwired: 9 in, 1 out]
          }
          frame 2 {
            n123 = Unbundle(w253) -> ("CtlRef"=w251:refnum<vi>, "Value"=w250:variant)
            n124 = Not A Number/Path/Refnum?(number/path/refnum=w251) -> (NaN/Path/Refnum?=w252:bool)
            n125 = case shown="False" w252 {
              tunnel: w251 -> [w256 _]
              tunnel: w250 -> [w255 _]
              frame False {
                # "Send a left mouse up"
                # "Reset the value"
                n126 = property class="Ctl"(reference=w256, "Val(Sgnl)"=w255) -> ()  [unwired: 1 in, 2 out]
                n127 = dll-call lib="user32.dll" fn="SendInput"("nInputs"=u32 1, "pInputs"=T14 {"type"=0, "KEYBDINPUT"={"dx"=0, "dy"=0, "mouseData"=0, "dwFlags"=4, "time"=0, "dwExtraInfo"=0}} ("input"), "cbSize"=u32 28) -> ()  [unwired: 7 in, 2 out]
              }
              frame True {
              }
            }
          }
        }
      }
      event Mouse Enter {
        w260 = FALSE ("Visible")
        n128 = event-data() -> ()  [unwired: 1 in, 4 out]
        n129 = property on="Deck1.DragDropPath" class="Path"("Visible"=w260) -> ()  [unwired: 2 in, 2 out]
        n130 = property on="Deck2.DragDropPath" class="Path"("Visible"=w260) -> ()  [unwired: 2 in, 2 out]
      }
      event Mouse Leave {
        w262 = TRUE ("Visible")
        n131 = event-data() -> ()  [unwired: 1 in, 4 out]
        n132 = property on="Deck1.DragDropPath" class="Path"("Visible"=w262) -> ()  [unwired: 2 in, 2 out]
        n133 = property on="Deck2.DragDropPath" class="Path"("Visible"=w262) -> ()  [unwired: 2 in, 2 out]
      }
    }
  }
  n134 = Unregister For Events(event registration refnum=w26) -> ()  [unwired: 1 in, 1 out]
  n135 = Release Queue(queue=w15, force destroy? (F)=TRUE, error in (no error)=w22) -> ()  [unwired: 3 out]
